vi "roi_points_extractor.vi"(10 "input cluster":T1) -> (2 "Points":i32[](array[numeric]))   [LabVIEW 2021]
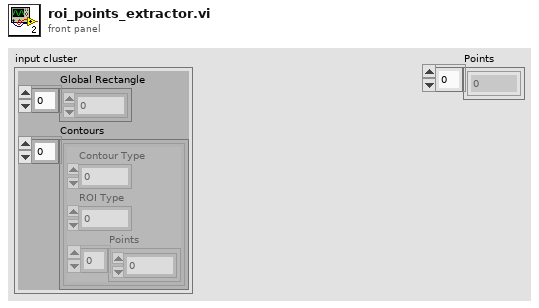
[diagram p1: front panel]
types:
  T1 = cluster{"Global Rectangle":i32[], "Contours":cluster{"Contour Type":u32, "ROI Type":u32, "Points":i32[]}[]}
  T2 = cluster{"Contour Type":u32, "ROI Type":u32, "Points":i32[]}[]
  T3 = cluster{"Contour Type":u32, "ROI Type":u32, "Points":i32[]}
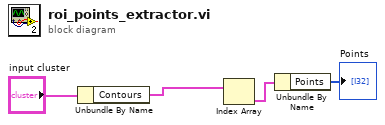
[diagram p0: block diagram]
diagram:
  n1 = Unbundle By Name("input cluster") -> ("Contours"=w4:T2)
  n2 = Index Array(array=w4) -> (element=w3:T3)  [unwired: 1 in]
  n3 = Unbundle By Name(w3) -> ("Points"=→"Points":i32[])
